vi "conv-var_vers_NUM.vi"(7 "Variable":string) -> (1 "Type Var. (Ch)":string, 2 "Num ?":bool, 3 "Type Var.":T1)   [LabVIEW 2010, in "lv_04.lvlib"]
uses:
  lv_04.lvlib
  commandes/c_enum_type_var.ctl
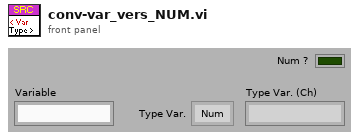
[diagram p1: front panel]
types:
  T1 = typedef "lv_04.lvlib/c_enum_type_var.ctl" = enum16{"Num", "Txt"}
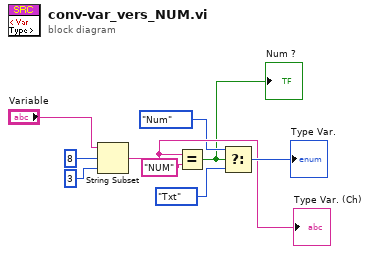
[diagram p0: block diagram]
diagram:
  n1 = String Subset(string="Variable", offset (0)=8, length (rest)=3 ("longueur (reste)")) -> (substring=w5:string)
  "Type Var. (Ch)" <- w5
  n2 = Equal?(x=w5, y="NUM") -> (x = y?=w1:bool)
  "Num ?" <- w1
  n3 = Select(t=c_enum_type_var."Num" ("Type Var."), s=w1, f=c_enum_type_var."Txt" ("Type Var.")) -> (s? t:f=→"Type Var.":T1)
